vi "Globals.vi"() -> ()   [LabVIEW 2009]
panel:
  in  "SaveInFile":bool
  in  "FileToSaveRefNum":refnum<file>
  in  "int32DeviceNumber":i32
  in  "FirmwareStringReady":bool
  in  "boolDeviceConnected":bool
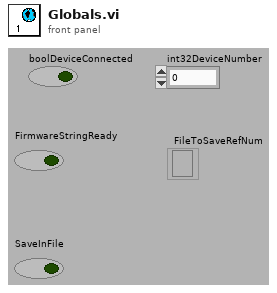
[diagram p1: front panel]
diagram:
